vi "Configure RemIO Module Core.vi"(8 "error in (no error)":errorcluster, 9 "module slot index":u8=1, 10 "Slave Ref In":refnum<k21>, 11 "11175 in":refnum<class "11175.lvclass">) -> (0 "error out":errorcluster, 1 "negative confirmation":T1 {"additional error code" format="%.0x"; "error code" format="%.0x"}, 2 "Slave Ref Out":refnum<k21>, 3 "11175 out":refnum<class "11175.lvclass">, 5 "SDO abort code":u32 format="%.0x")   [LabVIEW 2020, in "Modules.lvlib" / "11175.lvclass"]
uses:
  11175.lvclass
  <vilib>/indcomecat/Remote IO/typedefs/negative confirmation.ctl
  11175.lvclass/11175.ctl
  f93421cb-f380-4ccd-beff-48a1888eb290.vi
  RemIO Module/Get RemIO Library Path.vi
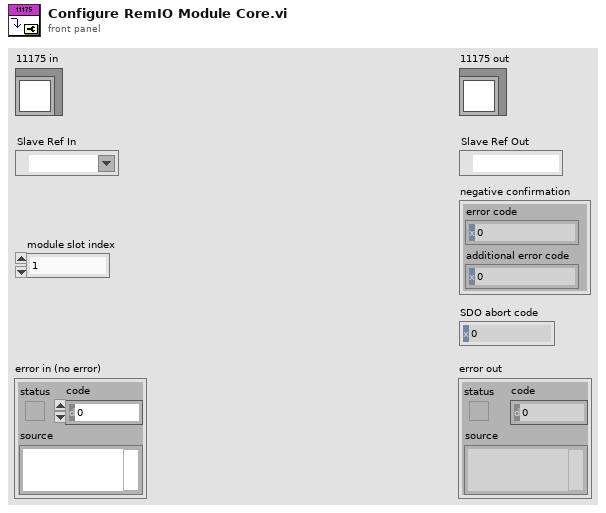
[diagram p1: front panel]
types:
  T1 = typedef "negative confirmation.ctl" = cluster{"error code":u16, "additional error code":u16}
  T2 = typedef "NI ECAT Remote IO.lvlib/subsititute value on error.ctl" = u8
  T3 = typedef "NI ECAT Remote IO.lvlib/report supply message.ctl" = u8
  T4 = cluster{"substitute value on error":T2, "report \"actuator supply not\npresent\" message?":T3}
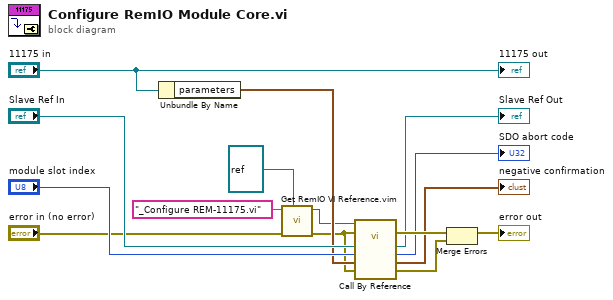
[diagram p0: block diagram]
diagram:
  n1 = Unbundle By Name("11175 in") -> ("parameters"=w6:T4)
  n2 = call "Get RemIO VI Reference.vim"("name or relative path"="_Configure REM-11175.vi", "error in (no error)"="error in (no error)", "type specifier VI Refnum (for type only)"=refnum<vi> refnum) -> ("vi reference"=w1:refnum<vi>, "error out"=w4:errorcluster)  [unwired: 6 in]
  n3 = call-by-ref "?"(reference=w1, error in=w4, 8:"error in (no error)"=w4, "parameters"=w6, "module slot index"="module slot index", "slave reference in"="Slave Ref In") -> (error out=w13:errorcluster, 0:"error out"=w14:errorcluster, "negative confirmation"=→"negative confirmation":T1, "SDO abort code"=→"SDO abort code":u32, "slave reference out"=→"Slave Ref Out":refnum<k21>)  [unwired: 4 in, 1 out]
  n4 = Merge Errors(w13, w14) -> (→"error out":errorcluster)
  "11175 out" <- "11175 in"
